vi "Draw Boundary Rectangle.vi"(10 "new picture in":picture, 11 "y":i16) -> (3 "new picture out":picture)   [LabVIEW 2015, in "LVJSON.lvlib" / "Shared.lvlib"]
uses:
  Shared.lvlib
  Get Object Parameters/offsets.vi
  Get Object Parameters/Get Object Parameters.xnode
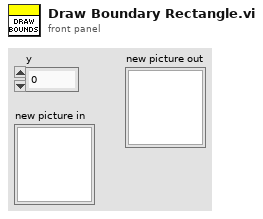
[diagram p1: front panel]
types:
  T1 = cluster{"left":i16, "top":i16, "right":i16, "bottom":i16}
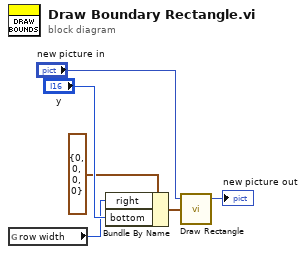
[diagram p0: block diagram]
diagram:
  n1 = global read "offsets.vi" "row width"() -> (w3:i16)
  n2 = Bundle By Name(cluster=T1 {"left"=0, "top"=0, "right"=0, "bottom"=0} ("rect"), "right"=w3, "bottom"="y") -> (w5:T1)
  n3 = call <vilib>:"Draw Rectangle.vi"("picture"="new picture in", "rect"=w5) -> ("new picture"=→"new picture out":picture)  [unwired: 7 in]
